vi "Write iSerialCommFactory.vi"(10 "ISerialCommFactory.lvclass":refnum<class "ISerialCommFactory.lvclass">, 11 "Model in":refnum<class "Model.lvclass">) -> (3 "Model out":refnum<class "Model.lvclass">)   [LabVIEW 2012, in "Model.lvclass"]
uses:
  Model.lvclass
  Program Files (x86)/National Instruments/LabVIEW 2012/user.lib/Common/SerialProtocols/SerialCommFactory/ISerialCommFactory/ISerialCommFactory.lvclass
  Model.lvclass/Model.ctl
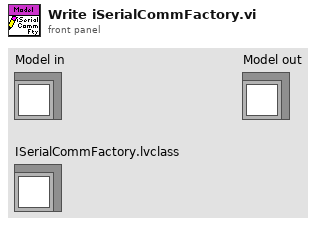
[diagram p1: front panel]
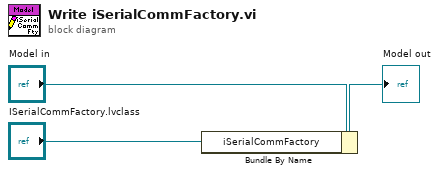
[diagram p0: block diagram]
diagram:
  n1 = Bundle By Name(cluster="Model in", "iSerialCommFactory"="ISerialCommFactory.lvclass") -> (→"Model out":refnum<class "Model.lvclass">)
